vi "lightsource-wl-correct.vi"(5 "PLE WL Input Cluster":T1={"WL Stepsize (nm)"=2, "WL Bandpass (nm)"=0, "Max WL VIS (nm)"=750, "Min WL VIS (nm)"=550} {"Min WL VIS (nm)" min=450 max=699 step=1; "Max WL VIS (nm)" min=501 max=850 step=1; "WL Bandpass (nm)" items=["5"=5, "10"=10, "25"=25, "50"=50, "75"=75, "100"=100]; "WL Stepsize (nm)" items=["5"=5, "10"=10, "25"=25, "50"=50, "75"=75, "100"=100]}) -> (1 "Output Cluster for While Loop":T2, 2 "PLE WL Output Cluster":T1={"WL Stepsize (nm)"=2, "WL Bandpass (nm)"=0, "Max WL VIS (nm)"=750, "Min WL VIS (nm)"=550} {"Min WL VIS (nm)" min=450 max=699 step=1; "Max WL VIS (nm)" min=501 max=850 step=1; "WL Bandpass (nm)" items=["5"=5, "10"=10, "25"=25, "50"=50, "75"=75, "100"=100]; "WL Stepsize (nm)" items=["5"=5, "10"=10, "25"=25, "50"=50, "75"=75, "100"=100]})   [LabVIEW 2017]
panel:
  # "Central Wavelength (nm)"
  # "Central Wavelength (nm)"
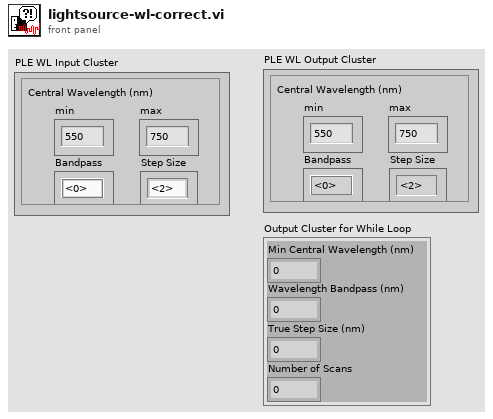
[diagram p1: front panel]
types:
  T1 = cluster{"WL Stepsize (nm)":i32, "WL Bandpass (nm)":u16, "Max WL VIS (nm)":i32, "Min WL VIS (nm)":i32}
  T2 = cluster{"Min Central Wavelength (nm)":i32, "Wavelength Bandpass (nm)":i32, "True Step Size (nm) ":i32, "Number of Scans":i32}
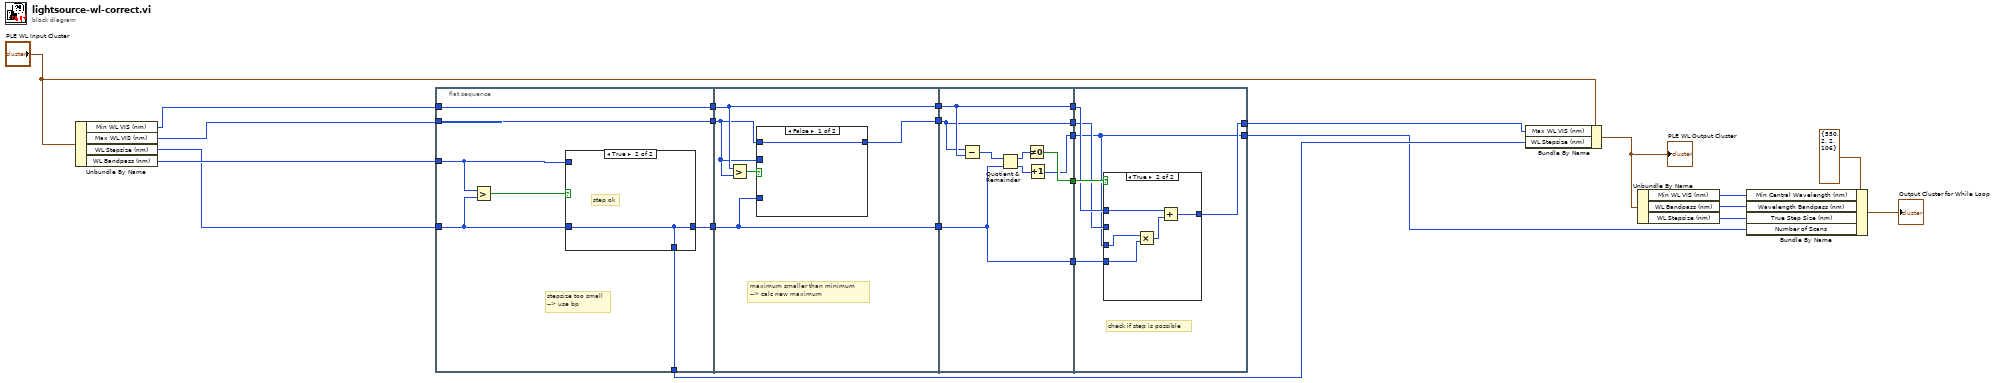
[diagram p0: block diagram]
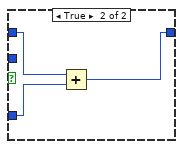
[diagram p3: hidden frame]
diagram:
  n1 = Unbundle By Name("PLE WL Input Cluster") -> ("Min WL VIS (nm)"=w15:i32, "Max WL VIS (nm)"=w14:i32, "WL Stepsize (nm)"=w24:i32, "WL Bandpass (nm)"=w25:u16)
  n2 = flat-sequence {
    tunnel: [w31] -> w13
    tunnel: [w28] -> w16
    tunnel: w24 -> [w32]
    tunnel: w25 -> [w30]
    tunnel: w15 -> [w27]
    tunnel: w14 -> [w26]
    tunnel: [w27] -> w11
    tunnel: [w26] -> w10
    tunnel: w13 -> [w37]
    tunnel: [w37] -> w12
    tunnel: w11 -> [w36]
    tunnel: w10 -> [w35]
    tunnel: [w38] -> w9
    tunnel: [w36] -> w8
    tunnel: w12 -> [w44]
    tunnel: w9 -> [w45]
    tunnel: w8 -> [w46]
    tunnel: [w47] -> w7
    tunnel: [w49] -> w6
    tunnel: [w46] -> w4
    tunnel: [w45] -> w3
    tunnel: [w44] -> w1
    tunnel: w7 -> [w52]
    tunnel: w6 -> [w57]
    tunnel: [w52] -> w5
    tunnel: w4 -> [w56]
    tunnel: w3 -> [w55]
    tunnel: [w54] -> w2
    tunnel: w1 -> [w53]
    frame #0 {
      # "stepsize too small\n--> use bp"
      n3 = Greater?(x=w30, y=w32) -> (0:w29:bool)
      n4 = case shown="True" w29 {
        tunnel: w32 -> [_ w34]
        tunnel: [w33 w34] -> w31
        tunnel: w30 -> [w33 _]
        tunnel: [w33 w34] -> w28
        frame False {
        }
        frame True {
          # "step ok"
        }
      }
    }
    frame #1 {
      # "maximum smaller than minimum\n--> calc new maximum"
      n5 = Greater?(x=w36, y=w35) -> (0:w39:bool)
      n6 = case shown="False" w39 {
        tunnel: w35 -> [w40 w42]
        tunnel: w35 -> [_ _]
        tunnel: [w40 w41] -> w38
        tunnel: w37 -> [_ w43]
        frame False {
        }
        frame True {
          n7 = Add(x=w42, y=w43) -> (x+y=w41:i32)
        }
      }
    }
    frame #2 {
      n8 = Subtract(x=w45, y=w46) -> (x-y=w50:i32)
      n9 = Quotient & Remainder(x=w50, y=w44) -> (x-y*floor(x/y)=w51:i32, floor(x/y)=w48:i32)
      n10 = Not Equal To 0?(x=w51) -> (x != 0?=w49:bool)
      n11 = Increment(x=w48) -> (x+1=w47:i32)
    }
    frame #3 {
      # "check if step is possible"
      n12 = case shown="True" w57 {
        tunnel: w56 -> [_ w63]
        tunnel: w55 -> [w58 _]
        tunnel: [w58 w59] -> w54
        tunnel: w53 -> [_ w62]
        tunnel: w52 -> [_ w61]
        frame False {
          # "clear cut"
        }
        frame True {
          n13 = Multiply(x=w61, y=w62) -> (x*y=w60:i32)
          n14 = Add(x=w63, y=w60) -> (x+y=w59:i32)
        }
      }
    }
  }
  n15 = Bundle By Name(cluster="PLE WL Input Cluster", "Max WL VIS (nm)"=w2, "WL Stepsize (nm)"=w16) -> (w20:T1)
  "PLE WL Output Cluster" <- w20
  n16 = Unbundle By Name(w20) -> ("Min WL VIS (nm)"=w19:i32, "WL Bandpass (nm)"=w18:u16, "WL Stepsize (nm)"=w17:i32)
  n17 = Bundle By Name(cluster=T2 {"Min Central Wavelength (nm)"=550, "Wavelength Bandpass (nm)"=2, "True Step Size (nm) "=2, "Number of Scans"=106} ("Output Cluster for While Loop"), "Min Central Wavelength (nm)"=w19, "Wavelength Bandpass (nm)"=w18, "True Step Size (nm)"=w17, "Number of Scans"=w5) -> (→"Output Cluster for While Loop":T2)
